vi "convert_strings.vi"(7 "Enum":T1, 8 "error in (no error)":errorcluster, 10 "BD Ring Text":string="\n\nPOS\n\nNEG\nACT\n", 11 "Instrument Command":string=":CALC:CHP:MARK:MODE %s;") -> (0 "error out":errorcluster, 2 "Disable String":string, 3 "Ring CMD/Enable String":string=":CALC:CHP:MARK:MODE POS;\r:CALC:CHP:MARK:MODE DELT;\r:CALC:CHP:MARK:MODE OFF;\r")   [LabVIEW 2018]
doc: "Converts raw command string to specific command string."
uses:
  TypeDefinitions/conver_strings_types.ctl
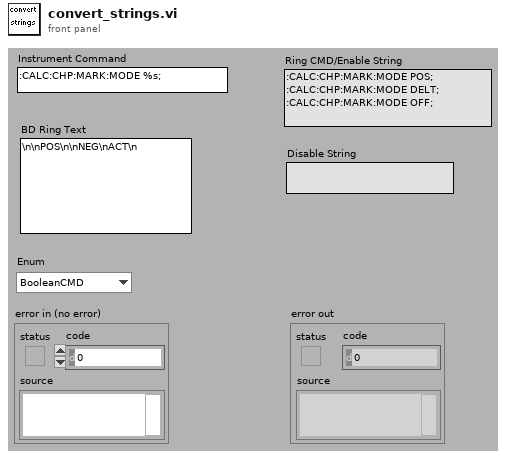
[diagram p1: front panel]
types:
  T1 = typedef "conver_strings_types.ctl" = enum16{"BooleanCMD", "RingCMD"}
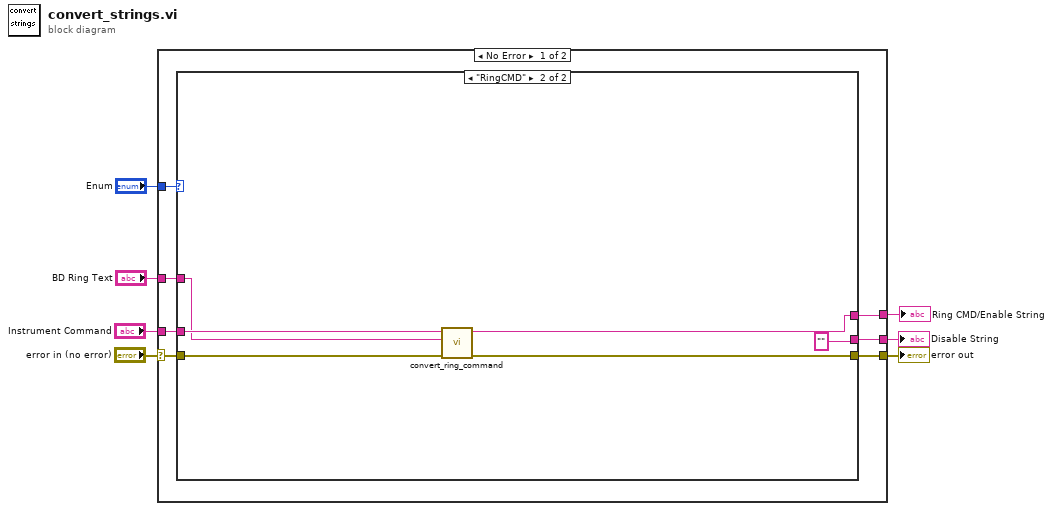
[diagram p0: block diagram]
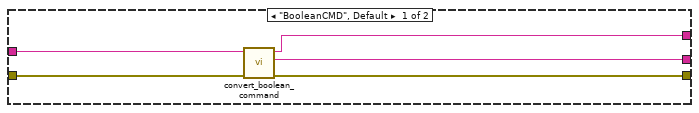
[diagram p2: hidden frame]
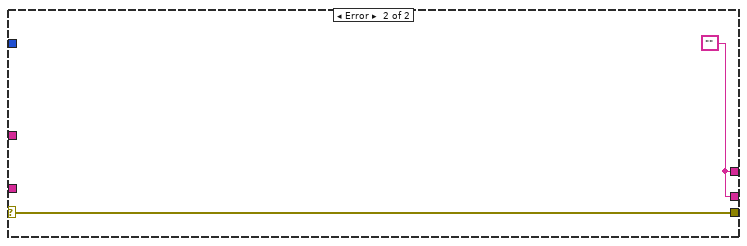
[diagram p3: hidden frame]
diagram:
  n1 = case shown="No Error" "error in (no error)" {
    selector: "error in (no error)" -> [w10 w27]
    tunnel: "Instrument Command" -> [w14 _]
    tunnel: [w13 w26] -> w6
    tunnel: "BD Ring Text" -> [w12 _]
    tunnel: [w9 w27] -> w3
    tunnel: "Enum" -> [w11 _]
    tunnel: [w8 w26] -> w1
    frame No Error {
      n2 = case shown="\"RingCMD\"" w11 {
        tunnel: w14 -> [w19 w24]
        tunnel: [w15 w20] -> w13
        tunnel: w12 -> [_ w23]
        tunnel: w10 -> [w18 w22]
        tunnel: [w17 w21] -> w9
        tunnel: [w16 "" ("result string")] -> w8
        frame "BooleanCMD", Default {
          n3 = call "convert_boolean_command.vi"("error in (no error)"=w18, "Instrument Command"=w19) -> ("error out"=w17:errorcluster, "DisableString"=w16:string, "EnableString"=w15:string)  [unwired: 7 out]
        }
        frame "RingCMD" {
          n4 = call "convert_ring_command.vi"("error in (no error)"=w22, "BD Ring Text"=w23, "Instrument Command"=w24) -> ("error out"=w21:errorcluster, "Ring CMD"=w20:string)  [unwired: 7 out]
        }
      }
    }
    frame Error {
      w26 = "" ("Instrument Command")
    }
  }
  "Ring CMD/Enable String" <- w6
  "error out" <- w3
  "Disable String" <- w1
